vi "DT_Triangle Manager_Find Connected Points.vi"(9 "base point idx":i32, 10 "triangle":i32, 11 "Triangles":i32[][](array[numeric])) -> (0 "error":i32, 1 "Connected Point Idx":i32[](array[numeric]), 2 "Connected Triangles":i32[](array[numeric]))   [LabVIEW 2020, in "NI_AAL_Geometry.lvlib"]
uses:
  <vilib>/Analysis/NI_AAL_Geometry.lvlib
  <vilib>/Analysis/geometry.llb/DT_Triangle Manager_Get Ghost Point.vi
  <vilib>/Analysis/geometry.llb/DT_Triangle Manager_Get Adj_by Point.vi
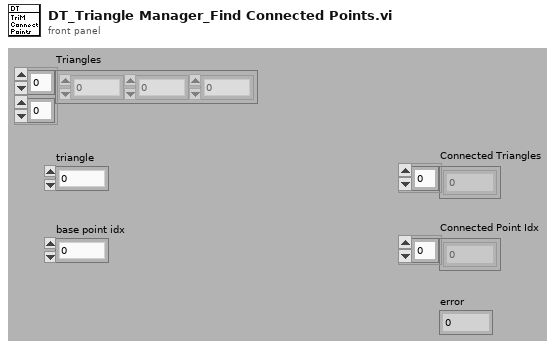
[diagram p1: front panel]
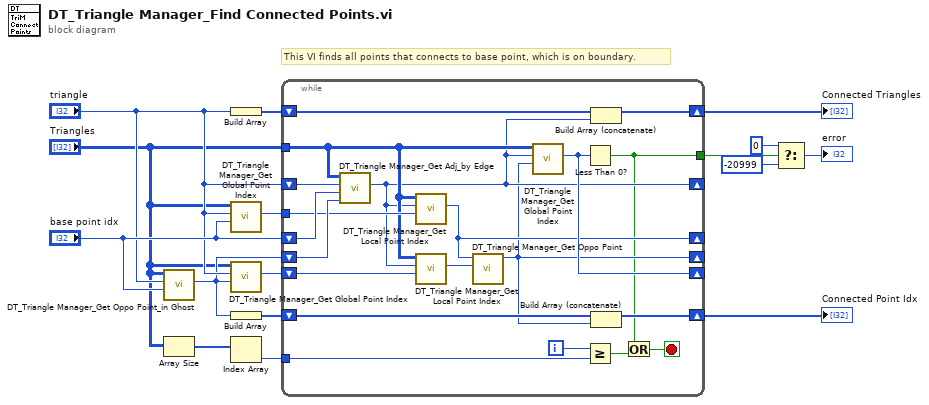
[diagram p0: block diagram]
diagram:
  # "This VI finds all points that connects to base point, which is on boundary."
  n1 = call <vilib>:"DT_Triangle Manager_Get Oppo Point_in Ghost.vi"("point idx"="base point idx", "triangle"="triangle", "Triangles"="Triangles") -> ("opposite point idx"=w11:i32)  [unwired: 8 out]
  n2 = Array Size(array="Triangles") -> (size(s)=w7:i32[])
  n3 = Build Array("triangle") -> (w12:i32[])
  n4 = call <vilib>:"DT_Triangle Manager_Get Global Point Index.vi"("local idx"="base point idx", "triangle"="triangle", "Triangles"="Triangles") -> ("global idx"=w16:i32)  [unwired: 8 out]
  n5 = call <vilib>:"DT_Triangle Manager_Get Global Point Index.vi"("local idx"=w11, "triangle"="triangle", "Triangles"="Triangles") -> ("global idx"=w15:i32)  [unwired: 8 out]
  n6 = Build Array(w11) -> (w10:i32[])
  n7 = Index Array(array=w7) -> (element=w5:i32)  [unwired: 1 in]
  n8 = while {
    shift-right: [w22] -> _
    shift-left: w11 -> [w34]
    shift-right: [w32] -> _
    shift-left: w15 -> [w31]
    shift-right: [w23] -> _
    shift-left: "triangle" -> [w35]
    tunnel: w16 -> [w33]
    shift-right: [w29] -> _
    shift-left: "base point idx" -> [w36]
    tunnel: "Triangles" -> [w28]
    shift-right: [w24] -> w9
    shift-left: w12 -> [w25]
    shift-right: [w26] -> w8
    shift-left: w10 -> [w27]
    tunnel: w5 -> [w20]
    tunnel: [w17] -> w2
    i -> [w21]
    stop <- w19 stop-if-true
    n9 = call <vilib>:"DT_Triangle Manager_Get Adj_by Edge.vi"("point idx 2"=w34, "point idx 1"=w36, "triangle"=w35, "Triangles"=w28) -> ("adj triangle"=w23:i32)  [unwired: 7 out]
    n10 = call <vilib>:"DT_Triangle Manager_Get Local Point Index.vi"("global idx"=w33, "triangle"=w23, "Triangles"=w28) -> ("local idx"=w29:i32)  [unwired: 8 out]
    n11 = call <vilib>:"DT_Triangle Manager_Get Local Point Index.vi"("global idx"=w31, "triangle"=w23, "Triangles"=w28) -> ("local idx"=w30:i32)  [unwired: 8 out]
    n12 = call <vilib>:"DT_Triangle Manager_Get Oppo Point.vi"("point idx 2"=w30, "point idx 1"=w29) -> ("oppo point idx"=w22:i32)  [unwired: 9 out]
    n13 = call <vilib>:"DT_Triangle Manager_Get Global Point Index.vi"("local idx"=w22, "triangle"=w23, "Triangles"=w28) -> ("global idx"=w32:i32)  [unwired: 8 out]
    n14 = Less Than 0?(x=w32) -> (x < 0?=w17:bool)
    n15 = Greater Or Equal?(x=w21, y=w20) -> (x >= y?=w18:bool)
    n16 = Build Array (concatenate)(w25, w23) -> (w24:i32[])
    n17 = Build Array (concatenate)(w27, w22) -> (w26:i32[])
    n18 = Or(x=w17, y=w18) -> (x .or. y?=w19:bool)
  }
  "Connected Triangles" <- w9
  "Connected Point Idx" <- w8
  n19 = Select(t=0, s=w2, f=-20999) -> (s? t:f=→"error":i32)
